vi "ConvertVerifyBoolToVerifyStr.vi"(11 "bool":bool) -> (3 "result":string)   [LabVIEW 2018, in "Library-DataConvert.lvlib"]
uses:
  Library-DataConvert.lvlib
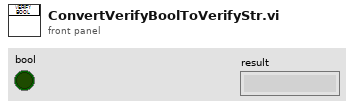
[diagram p1: front panel]
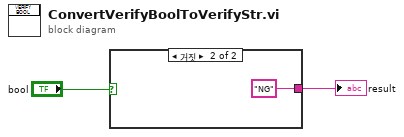
[diagram p0: block diagram]
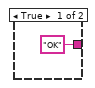
[diagram p2: hidden frame]
diagram:
  n1 = case shown="거짓" "bool" {
    tunnel: ["OK" "NG"] -> w1
    frame True {
    }
    frame False {
    }
  }
  "result" <- w1
